vi "计算纵横周中心坐标.vi"(11 "Center":cluster{"X":sgl, "Y":sgl}) -> (2 "所在直线 纵":sgl[](array[numeric]), 3 "所在直线 横":sgl[](array[numeric]))   [LabVIEW 2015]
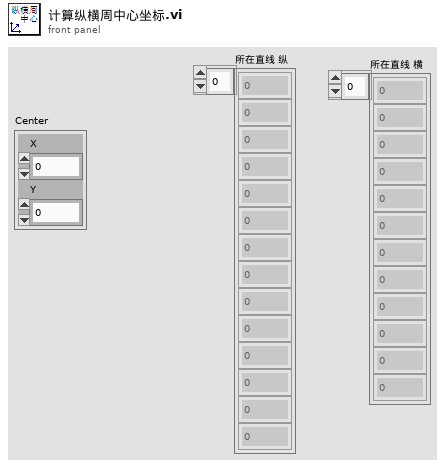
[diagram p1: front panel]
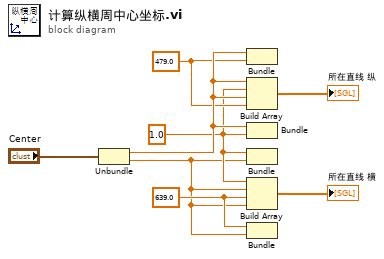
[diagram p0: block diagram]
diagram:
  w6 = sgl 639.0 ("element")
  w7 = sgl 479.0 ("element")
  w4 = sgl 1.0 ("element")
  n1 = Unbundle("Center") -> ("X"=w8:sgl, "Y"=w3:sgl)
  n2 = Bundle("X"=w8, "element"=w7) -> ()  [unwired: 1 in, 1 out]
  n3 = Build Array(w8, w4, w8, w7) -> (→"所在直线 纵":sgl[])
  n4 = Bundle("X"=w8, "element"=w4) -> ()  [unwired: 1 in, 1 out]
  n5 = Bundle("element"=w4, "Y"=w3) -> ()  [unwired: 1 in, 1 out]
  n6 = Build Array(w4, w3, w6, w3) -> (→"所在直线 横":sgl[])
  n7 = Bundle("element"=w6, "Y"=w3) -> ()  [unwired: 1 in, 1 out]
